vi "Log_FGV.vi"(7 "Log_mods":T1=enum."Write", 8 "error in":errorcluster, 11 "Log":string) -> (0 "error out":errorcluster)   [LabVIEW 2017]
uses:
  Log_mods.ctl
  Log_data.ctl
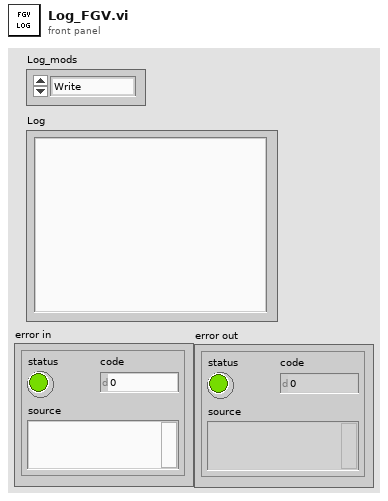
[diagram p1: front panel]
types:
  T1 = typedef "Log_mods.ctl" = enum16{"Init", "Write", "Clear", "End"}
  T2 = typedef "Log_data.ctl" = cluster{"VIRef":refnum<vi>, "RefLog":refnum<vi>, "Content":string, "Enabled":bool}
  T3 = enum32{"Invalid", "Standard", "Closed", "Hidden", "Minimized", "Maximized"}
  T4 = typedef "GameConfig_data.ctl" = cluster{"SpaceShip":cluster{"Angle":dbl, "SideLenght":dbl, "MaxLinearVeloc":dbl, "MaxAngularVeloc":dbl, "LinearAceleration":dbl, "AngularAceleration":dbl}, "Physics":cluster{"LinearDragFactor":dbl, "AngularDragFactor":dbl}, "Asteroids":cluster{"MaxSize":dbl, "MaxDivisions":i32, "MaxVeloc":dbl, "MinVeloc":dbl, "Fill":bool}, "Environment":cluster{"MaxAsteroids":i32, "TimeIncrement":dbl, "AsterProbCreation":dbl, "LogEnabled":bool}, "Shots":cluster{"MinTimeShots":dbl, "ShotSize":dbl, "ShotSpeed":dbl}}
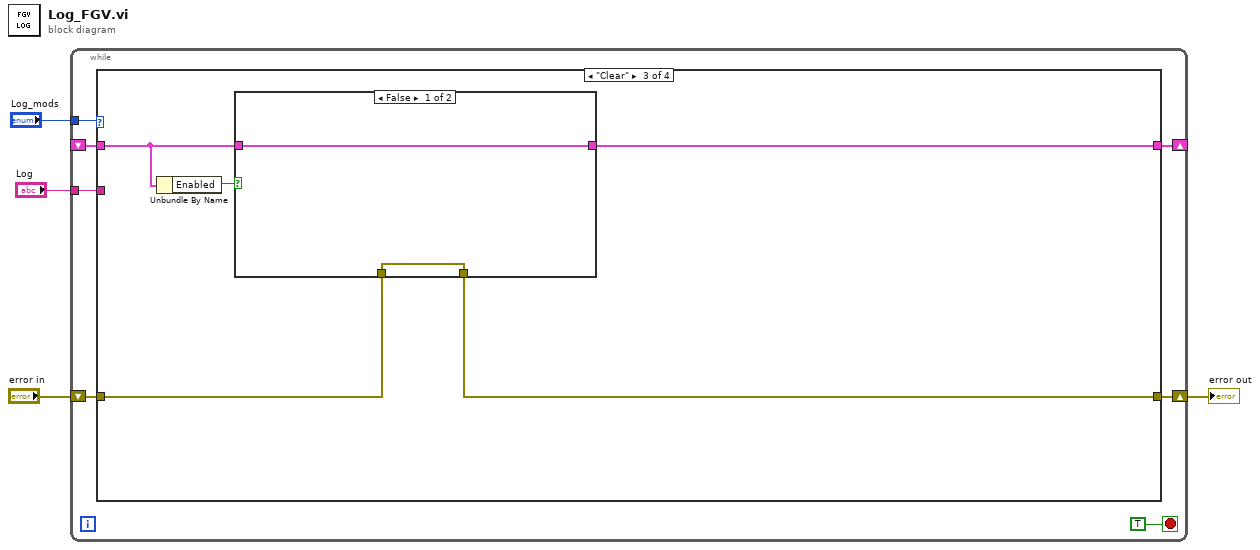
[diagram p0: block diagram]
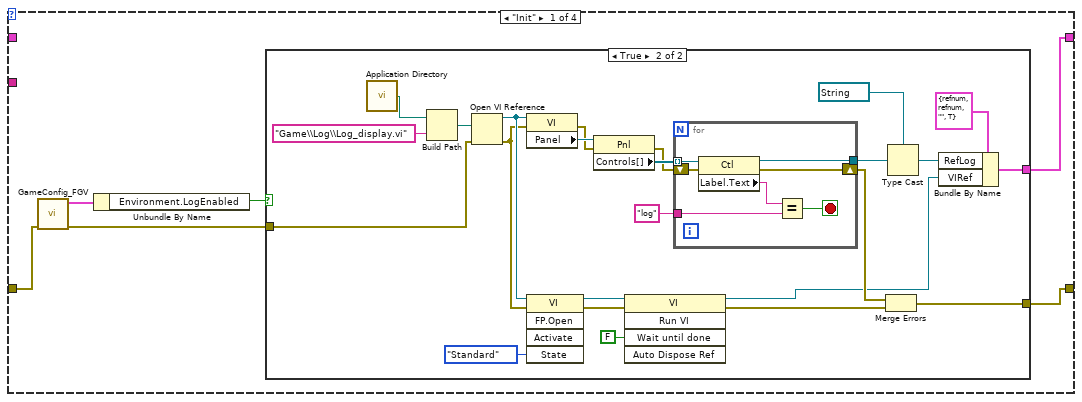
[diagram p2: hidden frame]
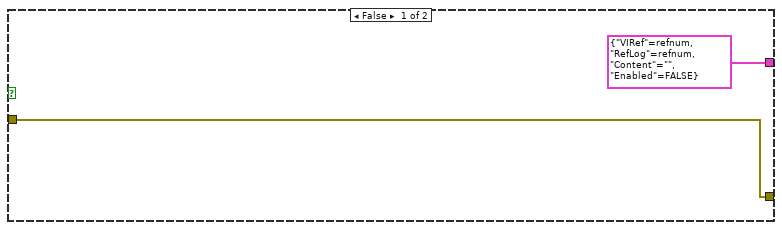
[diagram p3: hidden frame]
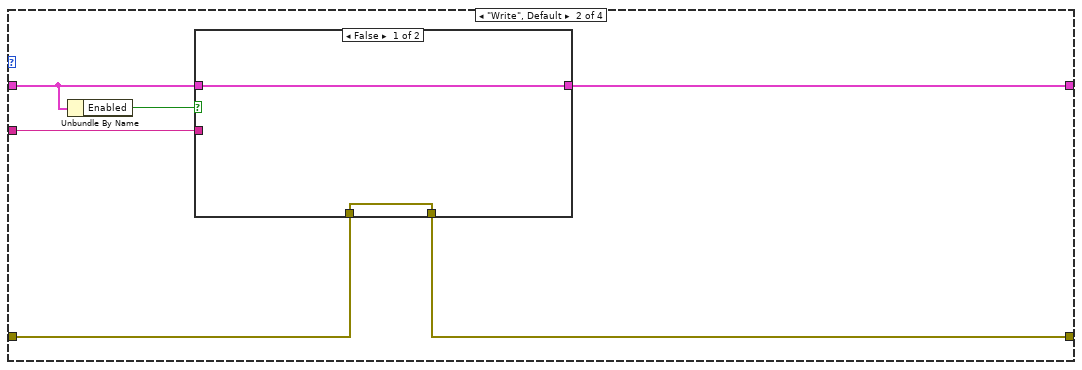
[diagram p4: hidden frame]
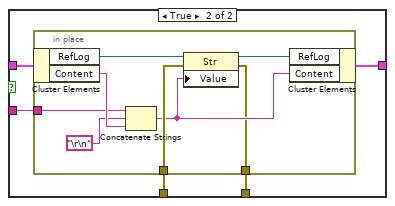
[diagram p5: hidden frame]
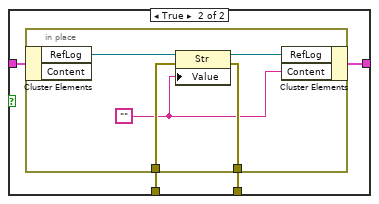
[diagram p6: hidden frame]
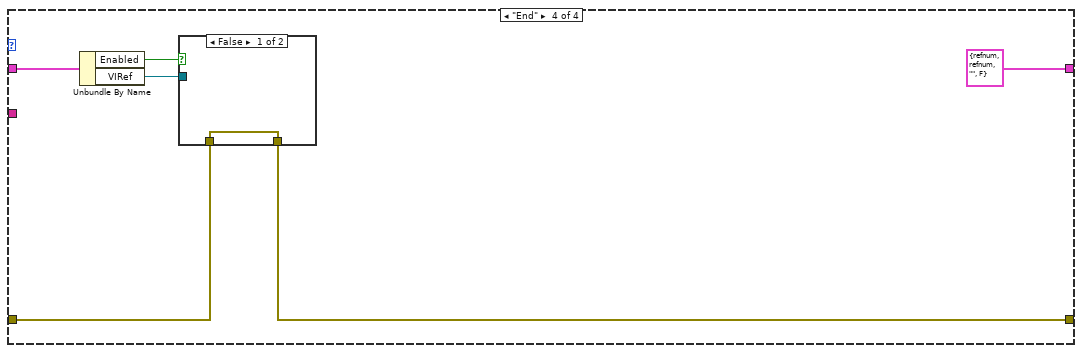
[diagram p7: hidden frame]
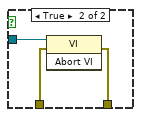
[diagram p8: hidden frame]
diagram:
  n1 = while {
    shift-right: [w8] -> w3
    shift-left: "error in" -> [w11]
    tunnel: "Log_mods" -> [w9]
    shift-right: [w7] -> _
    shift-left: _ -> [w6]
    tunnel: "Log" -> [w5]
    stop <- TRUE stop-if-true
    n2 = case shown="\"Clear\"" w9 {
      tunnel: w11 -> [w15 w55 w76 w91]
      tunnel: [w16 w54 w75 w90] -> w8
      tunnel: [w17 w53 w74 T2 {"VIRef"=refnum, "RefLog"=refnum, "Content"="", "Enabled"=FALSE} ("DataCluster")] -> w7
      tunnel: w6 -> [_ w52 w73 w93]
      tunnel: w5 -> [_ w56 _ _]
      frame "Init" {
        n3 = call "GameConfig_FGV.vi"("error in"=w15) -> ("error out"=w13:errorcluster, "Config"=w14:T4)  [unwired: 9 in]
        n4 = Unbundle By Name(w14) -> ("Environment.LogEnabled"=w12:bool)
        n5 = case shown="True" w12 {
          tunnel: [T2 {"VIRef"=refnum, "RefLog"=refnum, "Content"="", "Enabled"=FALSE} ("DataCluster") w23] -> w17
          tunnel: [w19 w22] -> w16
          tunnel: w13 -> [w19 w21]
          frame False {
          }
          frame True {
            n6 = call <vilib>:"Application Directory.vi"() -> ("Application Directory"=w43:path)
            n7 = Build Path(base path=w43, name or relative path="Game\\Log\\Log_display.vi") -> (appended path=w41:path)
            n8 = Open VI Reference(vi path=w41, error in (no error)=w21) -> (vi reference=w35:refnum<vi>, error out=w20:errorcluster)  [unwired: 4 in]
            n9 = property class="VI"(reference=w35, error in=w20) -> (error out=w39:errorcluster, "Panel"=w40:refnum<vi>)  [unwired: 1 out]
            n10 = invoke class="VI" method="FP.Open"(reference=w35, error in=w20, "State"=T3."Standard") -> (reference out=w34:refnum<vi>, error out=w33:errorcluster)  [unwired: 2 in, 3 out]
            n11 = property class="Pnl"(reference=w40, error in=w39) -> (error out=w37:errorcluster, "Controls[]"=w38:refnum<vi>[])  [unwired: 1 out]
            n12 = invoke class="VI" method="Run VI"(reference=w34, error in=w33, "Wait until done"=FALSE ("Wait Until Done")) -> (reference out=w24:refnum<vi>, error out=w30:errorcluster)  [unwired: 2 in, 3 out]
            n13 = for {
              tunnel: w38 -> [w50] mode=indexing
              shift-right: [w48] -> w29
              shift-left: w37 -> [w49]
              tunnel: "log" ("name or relative path") -> [w46]
              tunnel: [w44] -> w28
              stop <- w45 stop-if-true
              n14 = property class="Ctl"(reference=w50, error in=w49) -> (reference out=w44:refnum<vi>, error out=w48:errorcluster, "Label.Text"=w47:string)
              n15 = Equal?(x=w47, y=w46) -> (x = y?=w45:bool)
            }
            n16 = Merge Errors(w29, w30) -> (w22:errorcluster)
            n17 = Type Cast(type=refnum<vi> refnum ("RefLog"), x=w28) -> (*(type *) &x=w25:refnum<vi>)
            n18 = Bundle By Name(cluster=T2 {"VIRef"=refnum, "RefLog"=refnum, "Content"="", "Enabled"=TRUE} ("DataCluster"), "RefLog"=w25, "VIRef"=w24) -> (w23:T2)
          }
        }
      }
      frame "Write", Default {
        n19 = Unbundle By Name(w52) -> ("Enabled"=w51:bool)
        n20 = case shown="False" w51 {
          tunnel: w52 -> [w57 w63]
          tunnel: w56 -> [_ w62]
          tunnel: w55 -> [w58 w61]
          tunnel: [w58 w60] -> w54
          tunnel: [w57 w59] -> w53
          frame False {
          }
          frame True {
            n21 = in-place {
              in-place-border: w62 -> [w69]
              in-place-border: w61 -> [w71]
              in-place-border: [w64] -> w60
              n22 = in-place-cluster #1(w63) -> ("RefLog"=w67:refnum<vi>, "Content"=w70:string)
              n23 = Concatenate Strings(w69, "\r\n", w70) -> (w65:string)
              n24 = property class="Str"(reference=w67, error in=w71, "Value"=w65) -> (reference out=w66:refnum<vi>, error out=w64:errorcluster)
              n25 = in-place-cluster #1("RefLog"=w66, "Content"=w65) -> (w59:T2)
            }
          }
        }
      }
      frame "Clear" {
        n26 = Unbundle By Name(w73) -> ("Enabled"=w72:bool)
        n27 = case shown="False" w72 {
          tunnel: w73 -> [w77 w82]
          tunnel: w76 -> [w78 w81]
          tunnel: [w78 w80] -> w75
          tunnel: [w77 w79] -> w74
          frame False {
          }
          frame True {
            n28 = in-place {
              in-place-border: w81 -> [w87]
              in-place-border: [w84] -> w80
              w83 = ""
              n29 = in-place-cluster #2(w82) -> ("RefLog"=w86:refnum<vi>)  [unwired: 1 out]
              n30 = property class="Str"(reference=w86, error in=w87, "Value"=w83) -> (reference out=w85:refnum<vi>, error out=w84:errorcluster)
              n31 = in-place-cluster #2("RefLog"=w85, "Content"=w83) -> (w79:T2)
            }
          }
        }
      }
      frame "End" {
        n32 = Unbundle By Name(w93) -> ("Enabled"=w88:bool, "VIRef"=w92:refnum<vi>)
        n33 = case shown="False" w88 {
          tunnel: w92 -> [_ w97]
          tunnel: w91 -> [w94 w96]
          tunnel: [w94 w95] -> w90
          frame False {
          }
          frame True {
            n34 = invoke class="VI" method="Abort VI"(reference=w97, error in=w96) -> (error out=w95:errorcluster)  [unwired: 1 in, 2 out]
          }
        }
      }
    }
  }
  "error out" <- w3
